vi "Global Difficulty Level.vi"() -> ()   [LabVIEW 2020]
panel:
  in  "Difficulty Level":u8
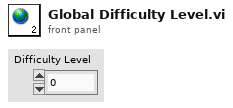
[diagram p1: front panel]
diagram:
